vi "test self.vi"() -> ()   [LabVIEW 2014]
uses:
  <vilib>/Utility/file.llb/Write To Spreadsheet File (DBL).vi
panel:
  out "XY Graph":cluster{"stage position out":dbl[], dbl[]}(graph)
  out "delta Xbead":dbl[](array[numeric])
  in  "X=T; Y=F":bool
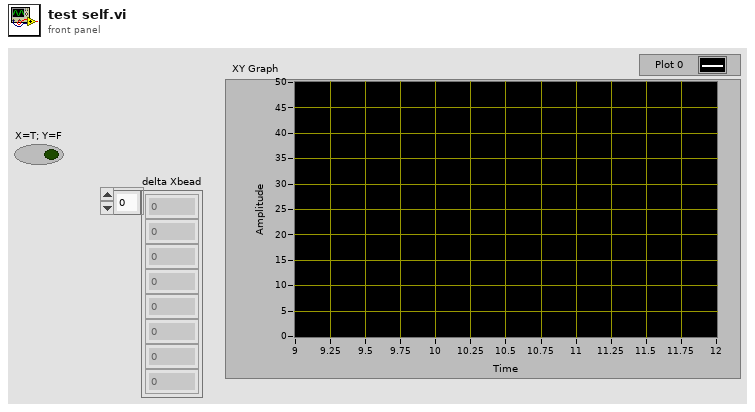
[diagram p1: front panel]
types:
  T1 = typedef "(1+2+3)fit stuckbead coefficient.ctl" = cluster{"(1)stuckbead-scan coefficient ":dbl[], "(2)stuckbead-scan coefficient ":dbl[], "(3)stuckbead-scan coefficient":dbl[]}
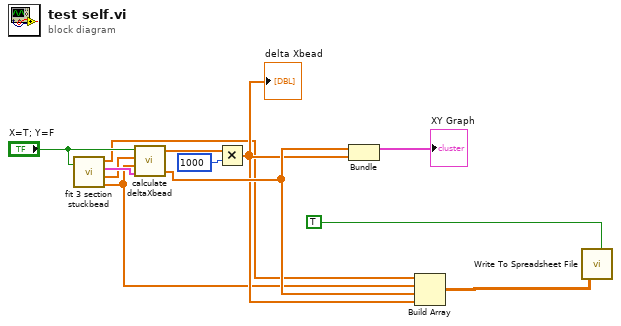
[diagram p0: block diagram]
diagram:
  n1 = call "fit 3 section stuckbead.vi"("X=T; Y=F"="X=T; Y=F") -> ("best fit position out"=w2:dbl[], "(1+2+3) stuckbead-scan coefficient"=w12:T1, "Calib-stage position (um)"=w10:dbl[], "Calib-QPD scan (V)"=w1:dbl[])  [unwired: 1 out]
  n2 = call "calculate deltaXbead.vi"("X=T; Y=F"="X=T; Y=F", "Stage position (um)"=w10, "QPD signal (V)"=w1, "(1+2+3) stuckbead-scan coefficient"=w12) -> ("delta Xbead (nm)"=w9:dbl[], "stage position out"=w5:dbl[])  [unwired: 2 in]
  n3 = Multiply(x=w9, y=1000) -> (x*y=w3:dbl[])
  "delta Xbead" <- w3
  n4 = Bundle("stage position out"=w5, w3) -> (→"XY Graph":cluster{"stage position out":dbl[], dbl[]})  [unwired: 1 in]
  n5 = Build Array(w2, w1, w5, w3) -> (w6:dbl[][])
  n6 = call-poly <vilib>:"Write To Spreadsheet File.vi"("transpose? (no:F)"=TRUE, "2D data"=w6) -> ()  [unwired: 6 in, 1 out]
